vi "2D Array 2 Cartesian Matrix.vi"(10 "Matrix In":dbl[][](array[numeric])) -> (2 "Matrix Out":T1)   [LabVIEW 2013]
uses:
  Metadata/Cartesian Matrix.ctl
  Metadata/Cartesian Point.ctl
  Metadata/Actuator Matrix.ctl
  Metadata/Actuator Point.ctl
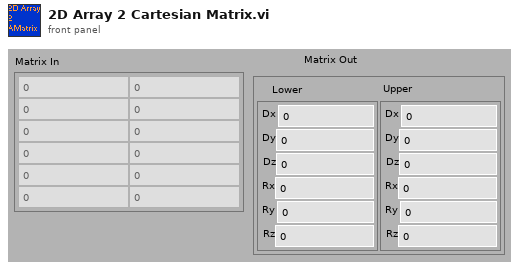
[diagram p1: front panel]
types:
  T1 = typedef "Cartesian Matrix.ctl" = cluster{"Lower":T2, "Upper":T2}
  T2 = typedef "Cartesian Point.ctl" = cluster{"Dx":dbl, "Dy":dbl, "Dz":dbl, "Rx":dbl, "Ry":dbl, "Rz":dbl}
  T3 = typedef "Actuator Matrix.ctl" = cluster{"Lower":T4, "Upper":T4}
  T4 = typedef "Actuator Point.ctl" = cluster{"X1":dbl, "X2":dbl, "Y1":dbl, "Z1":dbl, "Z2":dbl, "Z3":dbl}
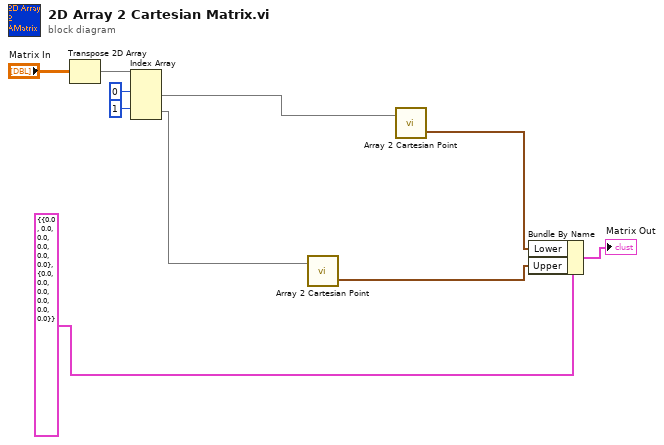
[diagram p0: block diagram]
diagram:
  n1 = Transpose 2D Array(2D array="Matrix In") -> (transposed array=w9:dbl[][])
  n2 = Index Array(array=w9, index (row) #1=0 ("index (row)"), index (row) #2=1 ("index (row)")) -> (element #1=w2:dbl[], element #2=w6:dbl[])  [unwired: 2 in]
  n3 = call "Array 2 Cartesian Point.vi"("Array"=w6) -> ("Cart Disp"=w3:T2)  [unwired: 2 in]
  n4 = call "Array 2 Cartesian Point.vi"("Array"=w2) -> ("Cart Disp"=w1:T2)  [unwired: 2 in]
  n5 = Bundle By Name(cluster=T3 {"Lower"={"X1"=0.0, "X2"=0.0, "Y1"=0.0, "Z1"=0.0, "Z2"=0.0, "Z3"=0.0}, "Upper"={"X1"=0.0, "X2"=0.0, "Y1"=0.0, "Z1"=0.0, "Z2"=0.0, "Z3"=0.0}} ("Matrix Out"), "Lower"=w1, "Upper"=w3) -> (→"Matrix Out":T3)
